vi "mainog_SEPERATELOOPS.vi"() -> ()   [LabVIEW 2014]
uses:
  <vilib>/Instr/_visa.llb/VISA Configure Serial Port (Instr).vi
panel:
  in  "stop":bool
  in  "Write Pressure Values 2":bool
  out "12bit DAC signal sent 2":string
  in  "Desired Pressures 2":dbl[](array[numeric])
  in  "Keep Data?":bool
  in  "filepath:":path
  out "Pressure Plot":i32[](graph)
  out "mbar":string[](array[string])
  out "status":bool
  out "error out":errorcluster
  in  "error in":errorcluster
  # "Arduino LabVIEW - Serial Read and Write"
  # "Measured Pressures"
  # "Desired pressures must be expressed in volts (0-5)"
  # "Channel 1"
  # "Channel 2"
  # "Channel 1"
  # "Channel 3"
  # "Channel 2"
  # "Channel 4"
  # "Channel 3"
  # "Channel 4"
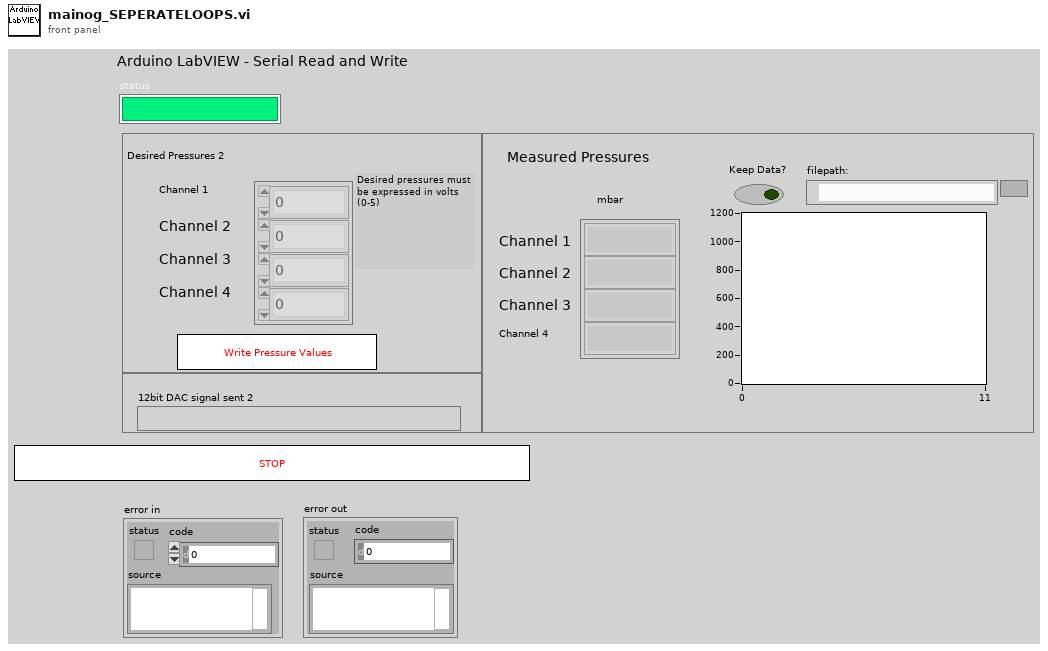
[diagram p1: front panel]
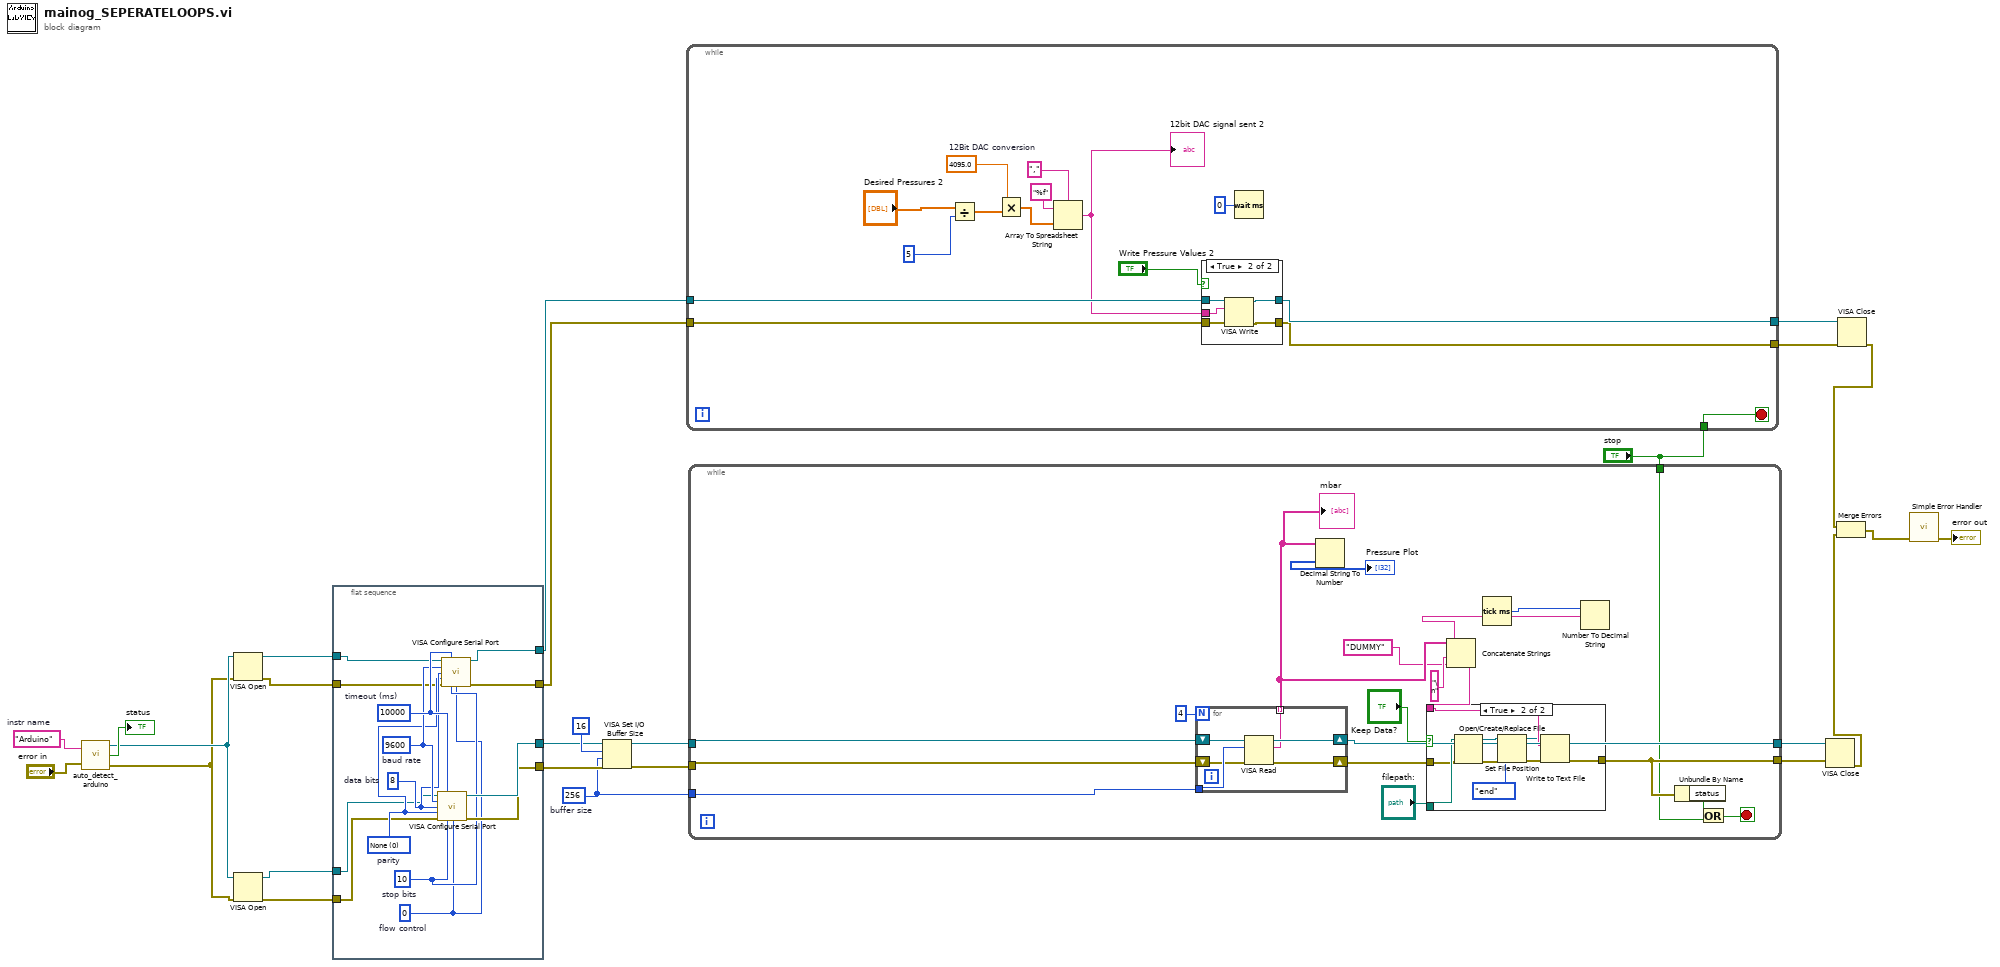
[diagram p0: block diagram]
diagram:
  w25 = "Arduino"  # instr name
  w19 = u32 256  # buffer size
  n1 = call "auto_detect_arduino.vi"("instr name"=w25, "error in"="error in") -> ("VISA resource name"=w14:refnum<visa-resource-name>, "status"=→"status":bool, "error out"=w13:errorcluster)
  n2 = VISA Open(error in (no error)=w13, VISA resource name=w14) -> (VISA resource name=w12:refnum<visa-resource-name>, error out=w11:errorcluster)  [unwired: 3 in]
  n3 = VISA Open(error in (no error)=w13, VISA resource name=w14) -> (VISA resource name=w10:refnum<visa-resource-name>, error out=w9:errorcluster)  [unwired: 3 in]
  n4 = flat-sequence {
    tunnel: [w40] -> w23
    tunnel: [w39] -> w22
    tunnel: w12 -> [w32]
    tunnel: w11 -> [w31]
    tunnel: w10 -> [w30]
    tunnel: w9 -> [w29]
    tunnel: [w28] -> w8
    tunnel: [w27] -> w7
    frame #0 {
      w33 = u16 0  # flow control
      w34 = u16 10  # stop bits
      w35 = u16 0 items=["None", "Odd", "Even", "Mark", "Space"]  # parity
      w36 = u16 8  # data bits
      w37 = u32 9600  # baud rate
      w38 = u32 10000  # timeout (ms)
      n5 = call-poly "VISA Configure Serial Port"("VISA resource name"=w30, "timeout (10sec)"=w38, "baud rate (9600)"=w37, "data bits (8)"=w36, "parity (0:none)"=w35, "error in (no error)"=w29, "stop bits (10: 1 bit)"=w34, "flow control (0:none)"=w33) -> ("VISA resource name out"=w40:refnum<visa-resource-name>, "error out"=w39:errorcluster)  [unwired: 6 in]
      n6 = call-poly "VISA Configure Serial Port"("VISA resource name"=w32, "timeout (10sec)"=w38, "baud rate (9600)"=w37, "data bits (8)"=w36, "parity (0:none)"=w35, "error in (no error)"=w31, "stop bits (10: 1 bit)"=w34, "flow control (0:none)"=w33) -> ("VISA resource name out"=w28:refnum<visa-resource-name>, "error out"=w27:errorcluster)  [unwired: 6 in]
    }
  }
  n7 = VISA Set I/O Buffer Size(VISA resource name=w23, mask (16)=u16 16 ("I/O Receive\nBuffer mask"), size (4096)=w19, error in (no error)=w22) -> (VISA resource name out=w21:refnum<visa-resource-name>, error out=w20:errorcluster)
  n8 = while {
    tunnel: w8 -> [w46]
    tunnel: w7 -> [w45]
    tunnel: [w43] -> w6
    tunnel: [w42] -> w5
    tunnel: "stop" -> [w41]
    stop <- w41 stop-if-true
    w49 = 4095.0  # 12Bit DAC conversion
    n9 = Divide(x="Desired Pressures 2", y=5) -> (x/y=w51:dbl[])
    n10 = Multiply(x=w49, y=w51) -> (x*y=w50:dbl[])
    n11 = Array To Spreadsheet String(delimiter (Tab)=",", array=w50, 3:"%f" ("format string")) -> (spreadsheet string=w44:string)
    "12bit DAC signal sent 2" <- w44
    n12 = case shown="True" "Write Pressure Values 2" {
      tunnel: w46 -> [w57 w62]
      tunnel: w45 -> [w56 w61]
      tunnel: [w57 w60] -> w43
      tunnel: [w56 w59] -> w42
      tunnel: w44 -> [_ w58]
      frame False {
      }
      frame True {
        n13 = VISA Write(VISA resource name=w62, write buffer=w58, error in (no error)=w61) -> (VISA resource name out=w60:refnum<visa-resource-name>, error out=w59:errorcluster)  [unwired: 1 out]
      }
    }
    n14 = Wait (ms)(milliseconds to wait=u32 0) -> ()  [unwired: 1 out]
  }
  n15 = while {
    tunnel: w21 -> [w66]
    tunnel: w20 -> [w65]
    tunnel: [w79] -> w26
    tunnel: w19 -> [w80]
    tunnel: [w74] -> w15
    tunnel: "stop" -> [w63]
    stop <- w81 stop-if-true
    n16 = for {
      N: 4 -> [_]
      tunnel: w80 -> [w96]
      tunnel: [w92] -> w67 mode=indexing
      shift-right: [w95] -> w79
      shift-left: w66 -> [w94]
      shift-right: [w97] -> w75
      shift-left: w65 -> [w93]
      n17 = VISA Read(VISA resource name=w94, byte count=w96, error in (no error)=w93) -> (VISA resource name out=w95:refnum<visa-resource-name>, read buffer=w92:string, error out=w97:errorcluster)  [unwired: 1 out]
    }
    "mbar" <- w67
    n18 = Decimal String To Number(string=w67) -> (number=→"Pressure Plot":i32[])  [unwired: 2 in, 1 out]
    n19 = Tick Count (ms)() -> (millisecond timer value=w68:u32)
    n20 = Number To Decimal String(number=w68) -> (decimal integer string=w69:string)  [unwired: 1 in]
    n21 = Concatenate Strings(w67, w69, "\n" ("string"), "DUMMY" ("string")) -> (w71:string)
    n22 = case shown="True" "Keep Data?" {
      tunnel: w71 -> [_ w91]
      tunnel: "filepath:" -> [_ w90]
      tunnel: w75 -> [w82 w89]
      tunnel: [w82 w84] -> w74
      frame False {
      }
      frame True {
        n23 = Open/Create/Replace File(file path (use dialog)=w90, error in=w89) -> (refnum out=w87:refnum<file>, error out=w88:errorcluster)  [unwired: 4 in, 1 out]
        n24 = Set File Position(refnum=w87, from (0:start)=enum16{"start", "end", "current"}."end", error in=w88) -> (refnum out=w86:refnum<file>, error out=w85:errorcluster)  [unwired: 1 in]
        n25 = Write to Text File(file (use dialog)=w86, text=w91, error in=w85) -> (error out=w84:errorcluster)  [unwired: 1 in, 2 out]
      }
    }
    n26 = Unbundle By Name(w74) -> ("status"=w73:bool)
    n27 = Or(x=w73, y=w63) -> (x .or. y?=w81:bool)
  }
  n28 = VISA Close(VISA resource name=w26, error in (no error)=w15) -> (error out=w3:errorcluster)
  n29 = VISA Close(VISA resource name=w6, error in (no error)=w5) -> (error out=w4:errorcluster)
  n30 = Merge Errors(w4, w3) -> (w2:errorcluster)
  n31 = call <vilib>:"Simple Error Handler.vi"("error in (no error)"=w2) -> ("error out"=→"error out":errorcluster)  [unwired: 4 in, 4 out]
